vi "Main VI.vi"() -> ()   [LabVIEW 2019]
uses:
  PhoneFromField/PhoneFromField.lvclass
panel:
  in  "Phone Number:":string
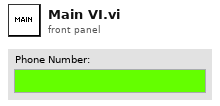
[diagram p1: front panel]
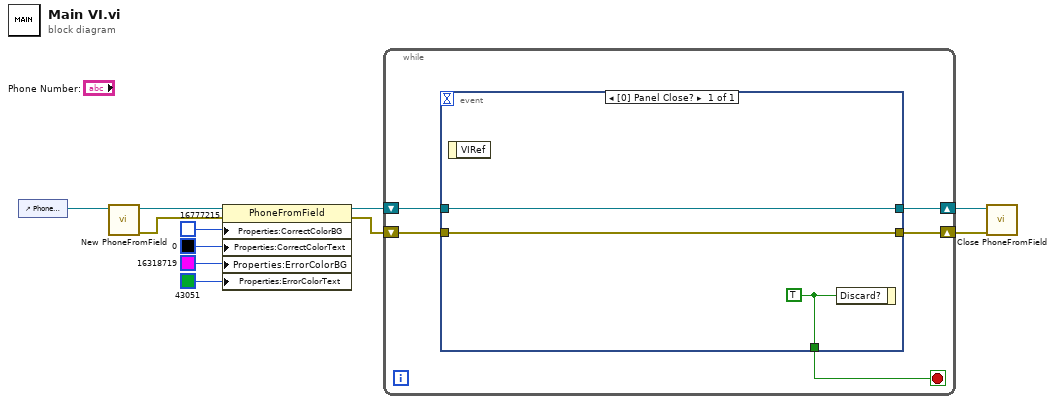
[diagram p0: block diagram]
diagram:
  n1 = control-ref of="Phone Number:"() -> (w10:refnum<vi>)
  n2 = call "New PhoneFromField.vi"("Reference"=w10) -> ("error out"=w11:errorcluster, "PhoneFromField out"=w6:refnum<class "PhoneFromField.lvclass">)  [unwired: 9 in]
  n3 = property class="PhoneFromField"(reference=w6, error in=w11, "Properties:CorrectColorBG"=u32 16777215 ("CorrectColorBG"), "Properties:CorrectColorText"=u32 0 ("CorrectColorText"), "Properties:ErrorColorBG"=u32 16318719 ("ErrorColorBG"), "Properties:ErrorColorText"=u32 43051 ("ErrorColorText")) -> (reference out=w5:refnum<class "PhoneFromField.lvclass">, error out=w7:errorcluster)
  n4 = while {
    shift-right: [w15] -> w9
    shift-left: w5 -> [w14]
    shift-right: [w13] -> w8
    shift-left: w7 -> [w12]
    stop <- w16 stop-if-true
    n5 = event shown="[0] Panel Close?" {
      selector: _ -> [_]
      dyn-events: _ -> [_]
      timeout: _ -> [_]
      tunnel: [w19] -> w16
      tunnel: [w18] -> w15
      tunnel: w14 -> [w18]
      tunnel: [w17] -> w13
      tunnel: w12 -> [w17]
      event Panel Close? {
        w19 = TRUE ("Discard?")
        n6 = event-data() -> ()  [unwired: 1 in, 1 out]
        n7 = event-data("Discard?"=w19) -> ()  [unwired: 1 in, 1 out]
      }
    }
  }
  n8 = call "Close PhoneFromField.vi"("error in (no error)"=w8, "PhoneFromField in"=w9) -> ()  [unwired: 9 in, 1 out]
